vi "Write and Read Configuration File.vi"() -> ()   [LabVIEW 2019]
doc: "JKI JSON 1.1.10.37\nTomi Maila - JKI\nCopyright (c) 2017, JKI"
uses:
  Classes/JSON Config File/JSON Config File.lvclass
panel:
  out "Configuration read from file":T1
  in  "Configuration to be saved to file":T1
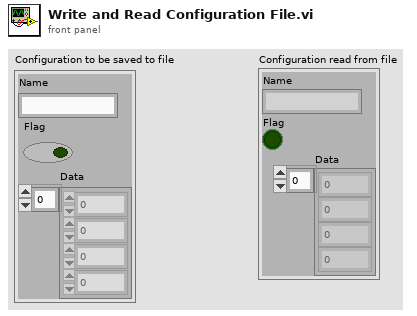
[diagram p1: front panel]
types:
  T1 = cluster{"Name":string, "Flag":bool, "Data":dbl[]}
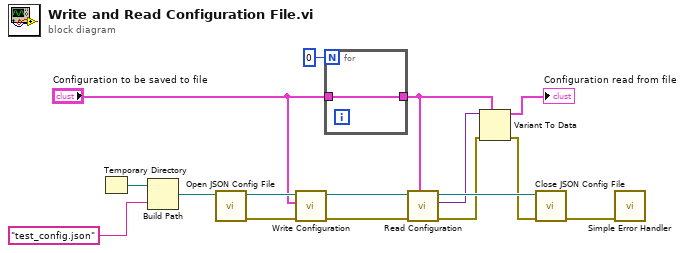
[diagram p0: block diagram]
diagram:
  n1 = Temporary Directory() -> (w16:path)
  n2 = Build Path(base path=w16, name or relative path="test_config.json") -> (appended path=w14:path)
  n3 = call "Open JSON Config File.vi"("Path"=w14) -> ("error out"=w12:errorcluster, "JSON Config File out"=w13:refnum<class "JSON Config File.lvclass">)  [unwired: 9 in]
  n4 = call-dynamic "Write Configuration.vi"("error in (no error)"=w12, "Configuration"="Configuration to be saved to file", "JSON Config File in"=w13) -> ("error out"=w10:errorcluster, "JSON Config File out"=w11:refnum<class "JSON Config File.lvclass">)  [unwired: 7 in]
  n5 = for {
    N: 0 -> [_]
    tunnel: [w17] -> w4
    tunnel: "Configuration to be saved to file" -> [w17]
  }
  n6 = call-dynamic "Read Configuration.vi"("Type and Defaults"=w4, "error in (no error)"=w10, "JSON Config File in"=w11) -> ("error out"=w3:errorcluster, "Configuration"=w5:variant, "JSON Config File out"=w9:refnum<class "JSON Config File.lvclass">)  [unwired: 6 in]
  n7 = Variant To Data(error in=w3, type=w4, Variant=w5) -> (data=→"Configuration read from file":T1, error out=w2:errorcluster)
  n8 = call-dynamic "Close JSON Config File.vi"("error in (no error)"=w2, "JSON Config File in"=w9) -> ("error out"=w8:errorcluster)  [unwired: 9 in]
  n9 = call <vilib>:"Simple Error Handler.vi"("error in (no error)"=w8) -> ()  [unwired: 4 in, 5 out]
